vi "U Boat decode controller.vi"(3 "Main sheet In":u16=1500, 4 "Jib Sheet In":u16=1500, 5 "Manual In":i32[](array[numeric])) -> (0 "Main sheet Out":u16, 1 "Rudder Out":u16=1500, 2 "Jib Steet Out":u16)   [LabVIEW 2013]
doc: "This VI takes in the axis information from a Logitech F310 Game controller and outputs the values for the Jib sheet, Main sheet, and Rudder servos."
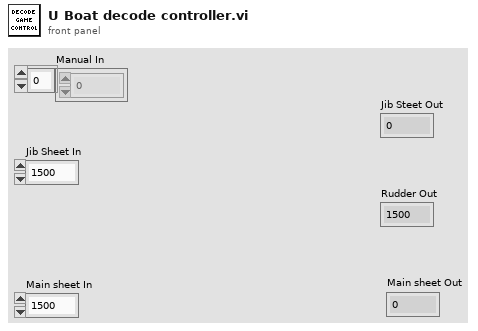
[diagram p1: front panel]
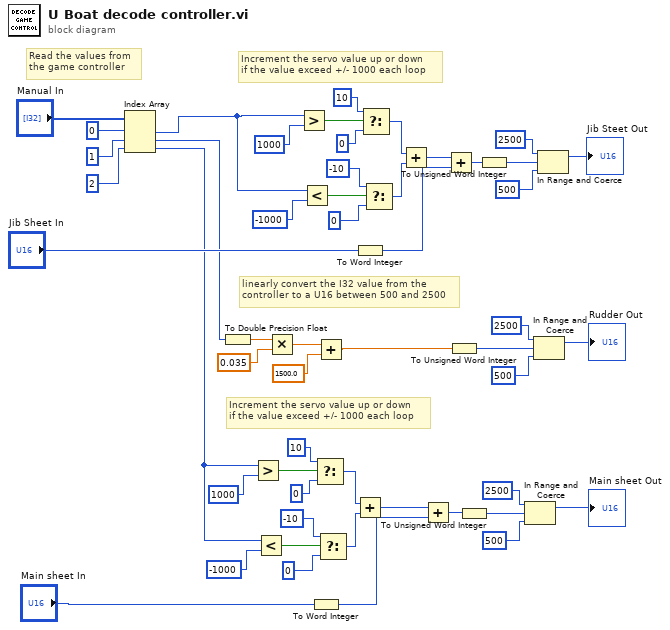
[diagram p0: block diagram]
diagram:
  # "Increment the servo value up or down\nif the value exceed +/- 1000 each loop"
  # "Read the values from\nthe game controller"
  # "Increment the servo value up or down\nif the value exceed +/- 1000 each loop"
  # "linearly convert the I32 value from the \ncontroller to a U16 between 500 and 2500"
  n1 = Index Array(array="Manual In", index #1=0 ("index"), index #2=1 ("index"), index #3=2 ("index")) -> (element #1=w16:i32, element #2=w15:i32, element #3=w14:i32)
  n2 = To Double Precision Float(number=w15) -> (double precision float=w52:dbl)
  n3 = Greater?(x=w14, y=1000) -> (0:w45:bool)
  n4 = Less?(x=w14, y=-1000) -> (x < y?=w41:bool)
  n5 = Multiply(x=w52, y=0.035) -> (x*y=w50:dbl)
  n6 = Greater?(x=w16, y=1000) -> (0:w27:bool)
  n7 = Less?(x=w16, y=-1000) -> (x < y?=w31:bool)
  n8 = To Word Integer(number="Main sheet In") -> (16bit integer=w37:i16)
  n9 = Select(t=i16 10, s=w45, f=i16 0) -> (s? t:f=w40:i16)
  n10 = Add(x=w50, y=1500.0) -> (x+y=w13:dbl)
  n11 = Select(t=i16 -10, s=w41, f=i16 0) -> (s? t:f=w39:i16)
  n12 = To Word Integer(number="Jib Sheet In") -> (16bit integer=w24:i16)
  n13 = Add(x=w40, y=w39) -> (x+y=w38:i16)
  n14 = Select(t=i16 10, s=w27, f=i16 0) -> (s? t:f=w32:i16)
  n15 = Select(t=i16 -10, s=w31, f=i16 0) -> (s? t:f=w33:i16)
  n16 = Add(x=w32, y=w33) -> (x+y=w34:i16)
  n17 = Add(x=w38, y=w37) -> (x+y=w36:i16)
  n18 = Add(x=w34, y=w24) -> (x+y=w35:i16)
  n19 = To Unsigned Word Integer(number=w13) -> (unsigned 16bit integer=w4:u16)
  n20 = To Unsigned Word Integer(number=w36) -> (unsigned 16bit integer=w2:u16)
  n21 = To Unsigned Word Integer(number=w35) -> (unsigned 16bit integer=w6:u16)
  n22 = In Range and Coerce(upper limit=u16 2500, x=w2, lower limit=u16 500) -> (coerced(x)=→"Main sheet Out":u16)  [unwired: 1 out]
  n23 = In Range and Coerce(upper limit=u16 2500, x=w4, lower limit=u16 500) -> (coerced(x)=→"Rudder Out":u16)  [unwired: 1 out]
  n24 = In Range and Coerce(upper limit=u16 2500, x=w6, lower limit=u16 500) -> (coerced(x)=→"Jib Steet Out":u16)  [unwired: 1 out]
